vi "sub_cmdparsing.vi"() -> ()   [LabVIEW 2017]
panel:
  in  "cmd":string
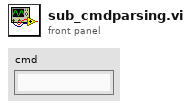
[diagram p1: front panel]
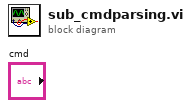
[diagram p0: block diagram]
diagram:
